vi "Replot.vi"(8 "error in (no error)":errorcluster, 11 "MagLabGraph in":refnum<class "XY Plot.lvclass">) -> (0 "error out":errorcluster, 3 "MagLabGraph out":refnum<class "XY Plot.lvclass">)   [LabVIEW 2016, in "XY Plot.lvclass"]
uses:
  XY Plot.lvclass
  D:/github/Measure_core/Plots/Plot/Plot.lvclass
  Plot/Plot.lvclass/Plot.ctl
  XY Plot.lvclass/XY Plot.ctl
  Plot/Read Data reduction.vi
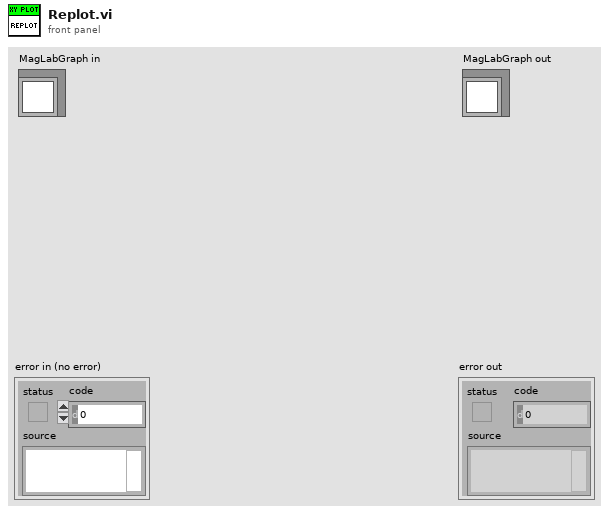
[diagram p1: front panel]
types:
  T1 = typedef "Data reduction.ctl" = cluster{"Clip time":bool, "Tiime 0":dbl, "Time 1":dbl, "Maximum data points":i32, "Decimation method":enum16{"coerce", "linear", "spline", "Min-Max", "Average"}}
  T2 = cluster{"File Path Control":path, "Group":string, "Channel":string, "Abbreviated":string}[]
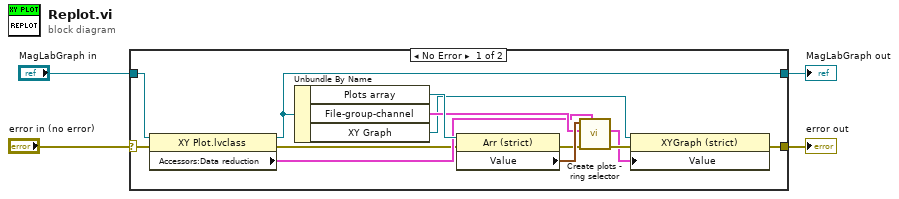
[diagram p0: block diagram]
diagram:
  n1 = case shown="No Error" "error in (no error)" {
    selector: "error in (no error)" -> [w5 w19]
    tunnel: [w12 w19] -> w1
    tunnel: [w8 w18] -> w2
    tunnel: "MagLabGraph in" -> [w17 w18]
    frame No Error {
      n2 = property class="XY Plot.lvclass"(reference=w17, error in=w5) -> (reference out=w8:refnum<class "XY Plot.lvclass">, error out=w6:errorcluster, "Accessors:Data reduction"=w7:T1)
      n3 = Unbundle By Name(w8) -> ("Plots array"=w16:refnum<vi>, "File-group-channel"=w14:T2, "XY Graph"=w11:refnum<vi>)
      n4 = property class="Arr (strict)"(reference=w16, error in=w6) -> (error out=w9:errorcluster, "Value"=w15:cluster{"X":u16, "Y":u16}[])  [unwired: 1 out]
      n5 = call "Create plots - ring selector.vi"("Data reduction"=w7, "Error In"=w9, "File-group-channel"=w14, "Plots  selector"=w15) -> ("Error Out"=w13:errorcluster, "Plots"=w10:cluster{dbl[], dbl[]}[])  [unwired: 6 in]
      n6 = property class="XYGraph (strict)"(reference=w11, error in=w13, "Value"=w10) -> (error out=w12:errorcluster)  [unwired: 1 out]
    }
    frame Error {
    }
  }
  "error out" <- w1
  "MagLabGraph out" <- w2
